vi "menuSelection.vi"(8 "error in (no error)":errorcluster, 9 "MenuRef":refnum<k9>, 10 "itemPath":string, 11 "ImageStreamViewer in":refnum<class "ImageStreamViewer.lvclass">) -> (0 "error out":errorcluster, 2 "close":bool, 3 "ImageStreamViewer out":refnum<class "ImageStreamViewer.lvclass">)   [LabVIEW 2011, in "Views.lvlib" / "Camera.lvlib" / "ImageStreamViewer.lvclass"]
uses:
  ImageStreamViewer.lvclass
  Tools/ImageProcessor/ImageAnalyser/AbsorptionAnalyser/AbsorptionAnalyser.lvclass
  Tools/ImageProcessor/ImageAnalyser/AbsorptionDS/AbsorptionDS.lvclass
  Tools/ImageProcessor/ImageAnalyser/FluorescenceAnalyser/FluorescenceAnalyser.lvclass
  Tools/ImageProcessor/ImageAnalyser/FluorescenceLiveAnalyser/FluorescenceLiveAnalyser.lvclass
  Tools/ImageProcessor/ImageAnalyser/TemperatureAnalyser/TemperatureAnalyser.lvclass
  Tools/ImageProcessor/ImageAnalyser/FringeTesting/FringeTesting.lvclass
  Tools/ImageProcessor/ImageAnalyser/Absorption2/Absorption2.lvclass
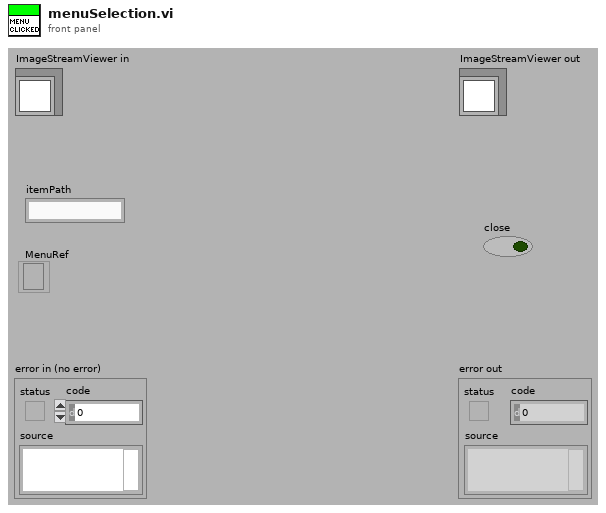
[diagram p1: front panel]
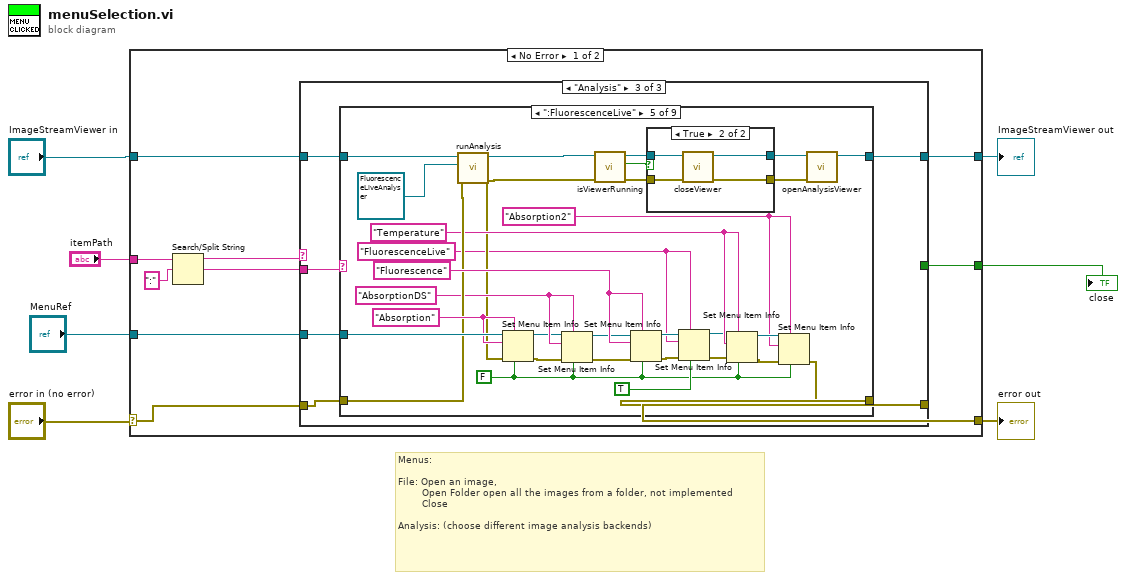
[diagram p0: block diagram]
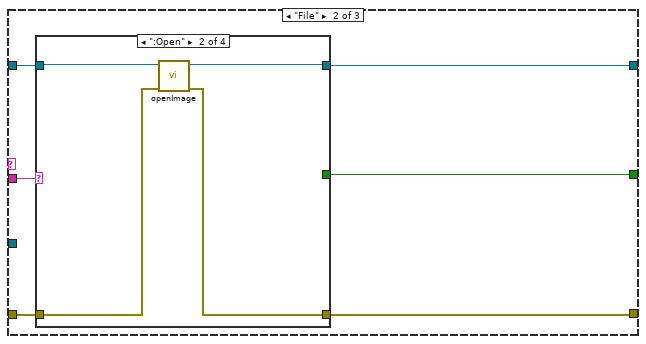
[diagram p3: hidden frame]
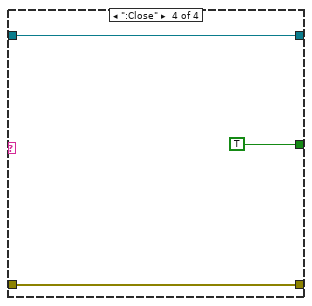
[diagram p6: hidden frame]
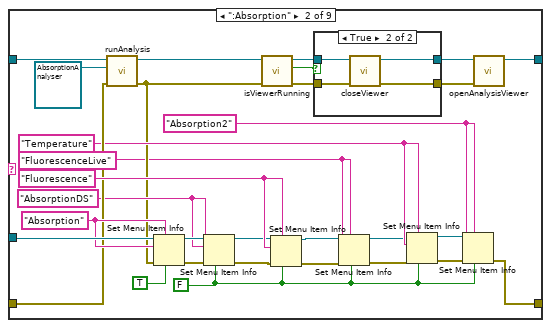
[diagram p8: hidden frame]
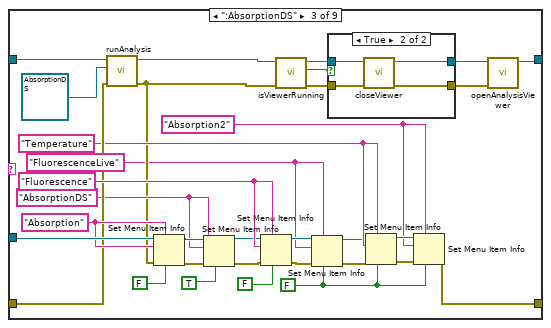
[diagram p10: hidden frame]
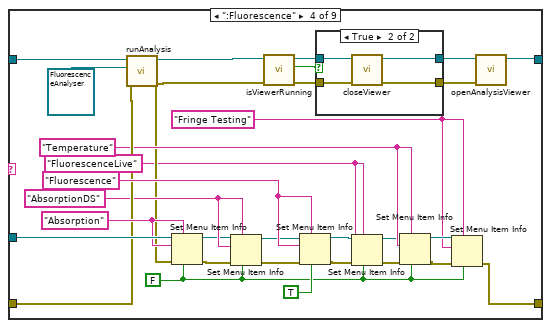
[diagram p12: hidden frame]
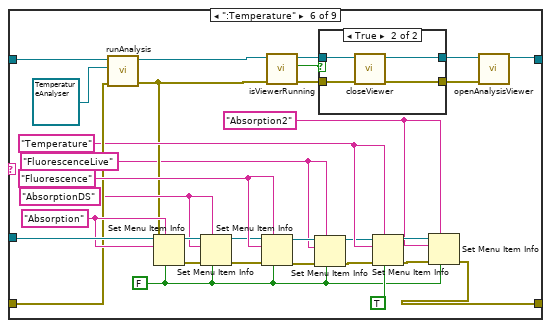
[diagram p15: hidden frame]
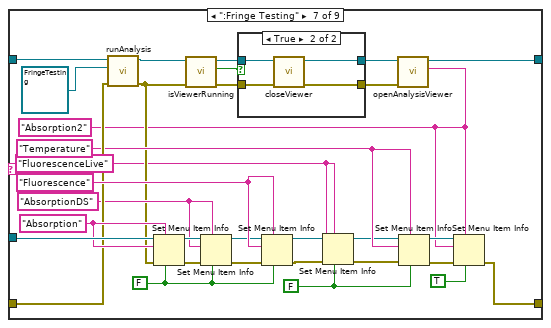
[diagram p17: hidden frame]
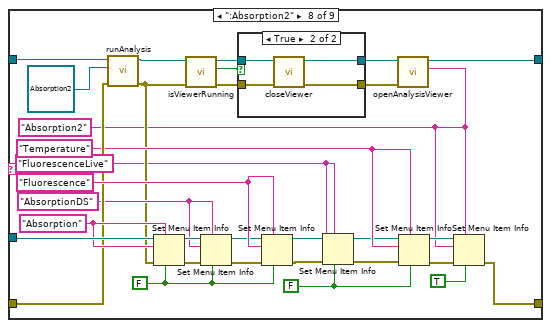
[diagram p19: hidden frame]
diagram:
  # "Menus: \n\nFile: Open an image, \n        Open Folder open all the images from a folder, not implemented\n        Close\n\nAnalysis: (choose different image analysis backends)"
  n1 = case shown="No Error" "error in (no error)" {
    selector: "error in (no error)" -> [w16 w313]
    tunnel: [w15 w313] -> w1
    tunnel: [w12 w312] -> w5
    tunnel: "ImageStreamViewer in" -> [w11 w312]
    tunnel: [w10 _] -> w6
    tunnel: "itemPath" -> [w9 _]
    tunnel: "MenuRef" -> [w8 _]
    frame No Error {
      n2 = Search/Split String(string=w9, search string/char (-)=":") -> (substring before match=w14:string, match + rest of string=w13:string)  [unwired: 1 in, 1 out]
      n3 = case shown="\"Analysis\"" w14 {
        tunnel: w16 -> [w18 w25 w39]
        tunnel: [w18 w24 w38] -> w15
        tunnel: w13 -> [_ w21 w40]
        tunnel: w11 -> [w19 w23 w42]
        tunnel: [w19 w22 w41] -> w12
        tunnel: [_ w20 _] -> w10
        tunnel: w8 -> [_ _ w37]
        frame Default {
        }
        frame "File" {
          n4 = case shown="\":Open\"" w21 {
            tunnel: w25 -> [w26 w29 w32 w35]
            tunnel: [w26 w28 w32 w35] -> w24
            tunnel: w23 -> [w27 w31 w33 w36]
            tunnel: [w27 w30 w33 w36] -> w22
            tunnel: [_ _ _ TRUE] -> w20
            frame Default {
            }
            frame ":Open" {
              n5 = call "openImage.vi"("error in (no error)"=w29, "ImageStreamViewer in"=w31) -> ("error out"=w28:errorcluster, "ImageStreamViewer out"=w30:refnum<class "ImageStreamViewer.lvclass">)  [unwired: 8 in]
            }
            frame ":Open Folder" {
            }
            frame ":Close" {
            }
          }
        }
        frame "Analysis" {
          n6 = case shown="\":FluorescenceLive\"" w40 {
            tunnel: w42 -> [w44 w71 w109 w148 w185 w222 w260 w298 w311]
            tunnel: [w44 w51 w88 w127 w166 w201 w239 w278 w310] -> w41
            tunnel: w39 -> [w43 w70 w108 w147 w184 w221 w259 w297 w309]
            tunnel: [w43 w59 w97 w136 w175 w210 w248 w286 w308] -> w38
            tunnel: w37 -> [_ w75 w114 w151 w188 w225 w263 w301 _]
            frame Default {
            }
            frame ":Absorption" {
              w46 = "FluorescenceLive"
              w60 = "Absorption2"
              w63 = "AbsorptionDS"
              w68 = "Temperature"
              w73 = "Absorption"
              w72 = "Fluorescence"
              w45 = FALSE
              n7 = call "runAnalysis.vi"("error in (no error)"=w70, "ImageAnalyser"=refnum<class "AbsorptionAnalyser.lvclass"> refnum ("Tools.lvlib:Imaging.lvlib:AbsorptionAnalyser.lvclass"), "ImageStreamViewer in"=w71) -> ("error out"=w52:errorcluster, "ImageStreamViewer out"=w53:refnum<class "ImageStreamViewer.lvclass">)  [unwired: 7 in]
              n8 = Set Menu Item Info(6:TRUE, 7:w73, 8:w52, 10:w73, 11:w75) -> (0:w65:errorcluster, 3:w67:refnum<k9>)  [unwired: 2 in]
              n9 = Set Menu Item Info(6:w45, 7:w63, 8:w65, 10:w63, 11:w67) -> (0:w64:errorcluster, 3:w66:refnum<k9>)  [unwired: 2 in]
              n10 = call "isViewerRunning.vi"("error in (no error)"=w52, "ImageStreamViewer in"=w53) -> ("error out"=w57:errorcluster, "running?"=w56:bool, "ImageStreamViewer out"=w58:refnum<class "ImageStreamViewer.lvclass">)  [unwired: 7 in]
              n11 = Set Menu Item Info(6:w45, 7:w72, 8:w64, 10:w72, 11:w66) -> (0:w48:errorcluster, 3:w50:refnum<k9>)  [unwired: 2 in]
              n12 = case shown="True" w56 {
                tunnel: w58 -> [w77 w81]
                tunnel: w57 -> [w76 w80]
                tunnel: [w77 w79] -> w55
                tunnel: [w76 w78] -> w54
                frame False {
                }
                frame True {
                  n13 = call "closeViewer.vi"("error in (no error)"=w80, "ImageStreamViewer in"=w81) -> ("error out"=w78:errorcluster, "ImageStreamViewer out"=w79:refnum<class "ImageStreamViewer.lvclass">)  [unwired: 8 in]
                }
              }
              n14 = Set Menu Item Info(6:w45, 7:w46, 8:w48, 10:w46, 11:w50) -> (0:w47:errorcluster, 3:w49:refnum<k9>)  [unwired: 2 in]
              n15 = Set Menu Item Info(6:w45, 7:w68, 8:w47, 10:w68, 11:w49) -> (0:w61:errorcluster, 3:w62:refnum<k9>)  [unwired: 2 in]
              n16 = Set Menu Item Info(6:w45, 7:w60, 8:w61, 10:w60, 11:w62) -> (0:w59:errorcluster)  [unwired: 2 in, 1 out]
              n17 = call "openAnalysisViewer.vi"("error in (no error)"=w54, "ImageStreamViewer in"=w55) -> ("ImageStreamViewer out"=w51:refnum<class "ImageStreamViewer.lvclass">)  [unwired: 8 in, 1 out]
            }
            frame ":AbsorptionDS" {
              w83 = "FluorescenceLive"
              w96 = "Absorption2"
              w100 = "AbsorptionDS"
              w107 = "Temperature"
              w82 = FALSE
              w111 = "Absorption"
              w110 = "Fluorescence"
              n18 = call "runAnalysis.vi"("error in (no error)"=w108, "ImageAnalyser"=refnum<class "AbsorptionDS.lvclass"> refnum ("Tools.lvlib:Imaging.lvlib:AbsorptionDS.lvclass"), "ImageStreamViewer in"=w109) -> ("error out"=w89:errorcluster, "ImageStreamViewer out"=w90:refnum<class "ImageStreamViewer.lvclass">)  [unwired: 7 in]
              n19 = Set Menu Item Info(6:FALSE, 7:w111, 8:w89, 10:w111, 11:w114) -> (0:w103:errorcluster, 3:w104:refnum<k9>)  [unwired: 2 in]
              n20 = Set Menu Item Info(6:TRUE, 7:w100, 8:w103, 10:w100, 11:w104) -> (0:w102:errorcluster, 3:w105:refnum<k9>)  [unwired: 2 in]
              n21 = Set Menu Item Info(6:FALSE, 7:w110, 8:w102, 10:w110, 11:w105) -> (0:w86:errorcluster, 3:w87:refnum<k9>)  [unwired: 2 in]
              n22 = call "isViewerRunning.vi"("error in (no error)"=w89, "ImageStreamViewer in"=w90) -> ("error out"=w94:errorcluster, "running?"=w93:bool, "ImageStreamViewer out"=w95:refnum<class "ImageStreamViewer.lvclass">)  [unwired: 7 in]
              n23 = Set Menu Item Info(6:w82, 7:w83, 8:w86, 10:w83, 11:w87) -> (0:w85:errorcluster, 3:w84:refnum<k9>)  [unwired: 2 in]
              n24 = case shown="True" w93 {
                tunnel: w95 -> [w116 w120]
                tunnel: w94 -> [w115 w119]
                tunnel: [w116 w118] -> w92
                tunnel: [w115 w117] -> w91
                frame False {
                }
                frame True {
                  n25 = call "closeViewer.vi"("error in (no error)"=w119, "ImageStreamViewer in"=w120) -> ("error out"=w117:errorcluster, "ImageStreamViewer out"=w118:refnum<class "ImageStreamViewer.lvclass">)  [unwired: 8 in]
                }
              }
              n26 = Set Menu Item Info(6:w82, 7:w107, 8:w85, 10:w107, 11:w84) -> (0:w98:errorcluster, 3:w99:refnum<k9>)  [unwired: 2 in]
              n27 = Set Menu Item Info(6:w82, 7:w96, 8:w98, 10:w96, 11:w99) -> (0:w97:errorcluster)  [unwired: 2 in, 1 out]
              n28 = call "openAnalysisViewer.vi"("error in (no error)"=w91, "ImageStreamViewer in"=w92) -> ("ImageStreamViewer out"=w88:refnum<class "ImageStreamViewer.lvclass">)  [unwired: 8 in, 1 out]
            }
            frame ":Fluorescence" {
              w121 = "FluorescenceLive"
              w135 = "Fringe Testing"
              w144 = "AbsorptionDS"
              w145 = "Temperature"
              w150 = "Absorption"
              w149 = "Fluorescence"
              w122 = FALSE
              n29 = call "runAnalysis.vi"("error in (no error)"=w147, "ImageAnalyser"=refnum<class "FluorescenceAnalyser.lvclass"> refnum ("Tools.lvlib:Imaging.lvlib:FluorescenceAnalyser.lvclass"), "ImageStreamViewer in"=w148) -> ("error out"=w128:errorcluster, "ImageStreamViewer out"=w129:refnum<class "ImageStreamViewer.lvclass">)  [unwired: 7 in]
              n30 = Set Menu Item Info(6:w122, 7:w150, 8:w128, 10:w150, 11:w151) -> (0:w141:errorcluster, 3:w143:refnum<k9>)  [unwired: 2 in]
              n31 = Set Menu Item Info(6:w122, 7:w144, 8:w141, 10:w144, 11:w143) -> (0:w140:errorcluster, 3:w142:refnum<k9>)  [unwired: 2 in]
              n32 = call "isViewerRunning.vi"("error in (no error)"=w128, "ImageStreamViewer in"=w129) -> ("error out"=w133:errorcluster, "running?"=w132:bool, "ImageStreamViewer out"=w134:refnum<class "ImageStreamViewer.lvclass">)  [unwired: 7 in]
              n33 = Set Menu Item Info(6:TRUE, 7:w149, 8:w140, 10:w149, 11:w142) -> (0:w123:errorcluster, 3:w126:refnum<k9>)  [unwired: 2 in]
              n34 = case shown="True" w132 {
                tunnel: w134 -> [w153 w157]
                tunnel: w133 -> [w152 w156]
                tunnel: [w153 w155] -> w131
                tunnel: [w152 w154] -> w130
                frame False {
                }
                frame True {
                  n35 = call "closeViewer.vi"("error in (no error)"=w156, "ImageStreamViewer in"=w157) -> ("error out"=w154:errorcluster, "ImageStreamViewer out"=w155:refnum<class "ImageStreamViewer.lvclass">)  [unwired: 8 in]
                }
              }
              n36 = Set Menu Item Info(6:w122, 7:w121, 8:w123, 10:w121, 11:w126) -> (0:w124:errorcluster, 3:w125:refnum<k9>)  [unwired: 2 in]
              n37 = Set Menu Item Info(6:w122, 7:w145, 8:w124, 10:w145, 11:w125) -> (0:w137:errorcluster, 3:w138:refnum<k9>)  [unwired: 2 in]
              n38 = Set Menu Item Info(6:w122, 7:w135, 8:w137, 10:w135, 11:w138) -> (0:w136:errorcluster)  [unwired: 2 in, 1 out]
              n39 = call "openAnalysisViewer.vi"("error in (no error)"=w130, "ImageStreamViewer in"=w131) -> ("ImageStreamViewer out"=w127:refnum<class "ImageStreamViewer.lvclass">)  [unwired: 8 in, 1 out]
            }
            frame ":FluorescenceLive" {
              w160 = "FluorescenceLive"
              w174 = "Absorption2"
              w182 = "AbsorptionDS"
              w183 = "Temperature"
              w187 = "Absorption"
              w186 = "Fluorescence"
              w158 = FALSE
              n40 = call "runAnalysis.vi"("error in (no error)"=w184, "ImageAnalyser"=refnum<class "FluorescenceLiveAnalyser.lvclass"> refnum ("Tools.lvlib:Imaging.lvlib:FluorescenceLiveAnalyser.lvclass"), "ImageStreamViewer in"=w185) -> ("error out"=w167:errorcluster, "ImageStreamViewer out"=w168:refnum<class "ImageStreamViewer.lvclass">)  [unwired: 7 in]
              n41 = Set Menu Item Info(6:w158, 7:w187, 8:w167, 10:w187, 11:w188) -> (0:w179:errorcluster, 3:w181:refnum<k9>)  [unwired: 2 in]
              n42 = Set Menu Item Info(6:w158, 7:w182, 8:w179, 10:w182, 11:w181) -> (0:w178:errorcluster, 3:w180:refnum<k9>)  [unwired: 2 in]
              n43 = call "isViewerRunning.vi"("error in (no error)"=w167, "ImageStreamViewer in"=w168) -> ("error out"=w172:errorcluster, "running?"=w171:bool, "ImageStreamViewer out"=w173:refnum<class "ImageStreamViewer.lvclass">)  [unwired: 7 in]
              n44 = Set Menu Item Info(6:w158, 7:w186, 8:w178, 10:w186, 11:w180) -> (0:w163:errorcluster, 3:w164:refnum<k9>)  [unwired: 2 in]
              n45 = case shown="True" w171 {
                tunnel: w173 -> [w190 w194]
                tunnel: w172 -> [w189 w193]
                tunnel: [w190 w192] -> w170
                tunnel: [w189 w191] -> w169
                frame False {
                }
                frame True {
                  n46 = call "closeViewer.vi"("error in (no error)"=w193, "ImageStreamViewer in"=w194) -> ("error out"=w191:errorcluster, "ImageStreamViewer out"=w192:refnum<class "ImageStreamViewer.lvclass">)  [unwired: 8 in]
                }
              }
              n47 = Set Menu Item Info(6:TRUE, 7:w160, 8:w163, 10:w160, 11:w164) -> (0:w162:errorcluster, 3:w161:refnum<k9>)  [unwired: 2 in]
              n48 = Set Menu Item Info(6:w158, 7:w183, 8:w162, 10:w183, 11:w161) -> (0:w176:errorcluster, 3:w177:refnum<k9>)  [unwired: 2 in]
              n49 = Set Menu Item Info(6:w158, 7:w174, 8:w176, 10:w174, 11:w177) -> (0:w175:errorcluster)  [unwired: 2 in, 1 out]
              n50 = call "openAnalysisViewer.vi"("error in (no error)"=w169, "ImageStreamViewer in"=w170) -> ("ImageStreamViewer out"=w166:refnum<class "ImageStreamViewer.lvclass">)  [unwired: 8 in, 1 out]
            }
            frame ":Temperature" {
              w196 = "FluorescenceLive"
              w209 = "Absorption2"
              w213 = "AbsorptionDS"
              w219 = "Temperature"
              w224 = "Absorption"
              w223 = "Fluorescence"
              w195 = FALSE
              n51 = call "runAnalysis.vi"("error in (no error)"=w221, "ImageAnalyser"=refnum<class "TemperatureAnalyser.lvclass"> refnum ("Tools.lvlib:Imaging.lvlib:TemperatureAnalyser.lvclass"), "ImageStreamViewer in"=w222) -> ("error out"=w202:errorcluster, "ImageStreamViewer out"=w203:refnum<class "ImageStreamViewer.lvclass">)  [unwired: 7 in]
              n52 = Set Menu Item Info(6:w195, 7:w224, 8:w202, 10:w224, 11:w225) -> (0:w215:errorcluster, 3:w217:refnum<k9>)  [unwired: 2 in]
              n53 = Set Menu Item Info(6:w195, 7:w213, 8:w215, 10:w213, 11:w217) -> (0:w214:errorcluster, 3:w216:refnum<k9>)  [unwired: 2 in]
              n54 = Set Menu Item Info(6:w195, 7:w223, 8:w214, 10:w223, 11:w216) -> (0:w197:errorcluster, 3:w200:refnum<k9>)  [unwired: 2 in]
              n55 = call "isViewerRunning.vi"("error in (no error)"=w202, "ImageStreamViewer in"=w203) -> ("error out"=w207:errorcluster, "running?"=w206:bool, "ImageStreamViewer out"=w208:refnum<class "ImageStreamViewer.lvclass">)  [unwired: 7 in]
              n56 = Set Menu Item Info(6:w195, 7:w196, 8:w197, 10:w196, 11:w200) -> (0:w198:errorcluster, 3:w199:refnum<k9>)  [unwired: 2 in]
              n57 = case shown="True" w206 {
                tunnel: w208 -> [w227 w231]
                tunnel: w207 -> [w226 w230]
                tunnel: [w227 w229] -> w205
                tunnel: [w226 w228] -> w204
                frame False {
                }
                frame True {
                  n58 = call "closeViewer.vi"("error in (no error)"=w230, "ImageStreamViewer in"=w231) -> ("error out"=w228:errorcluster, "ImageStreamViewer out"=w229:refnum<class "ImageStreamViewer.lvclass">)  [unwired: 8 in]
                }
              }
              n59 = Set Menu Item Info(6:TRUE, 7:w219, 8:w198, 10:w219, 11:w199) -> (0:w211:errorcluster, 3:w212:refnum<k9>)  [unwired: 2 in]
              n60 = Set Menu Item Info(6:w195, 7:w209, 8:w211, 10:w209, 11:w212) -> (0:w210:errorcluster)  [unwired: 2 in, 1 out]
              n61 = call "openAnalysisViewer.vi"("error in (no error)"=w204, "ImageStreamViewer in"=w205) -> ("ImageStreamViewer out"=w201:refnum<class "ImageStreamViewer.lvclass">)  [unwired: 8 in, 1 out]
            }
            frame ":Fringe Testing" {
              w233 = "FluorescenceLive"
              w238 = "Absorption2"
              w252 = "AbsorptionDS"
              w232 = FALSE
              w258 = "Temperature"
              w262 = "Absorption"
              w261 = "Fluorescence"
              w253 = FALSE
              n62 = call "runAnalysis.vi"("error in (no error)"=w259, "ImageAnalyser"=refnum<class "FringeTesting.lvclass"> refnum ("Tools.lvlib:Imaging.lvlib:FringeTesting.lvclass"), "ImageStreamViewer in"=w260) -> ("error out"=w245:errorcluster, "ImageStreamViewer out"=w246:refnum<class "ImageStreamViewer.lvclass">)  [unwired: 7 in]
              n63 = Set Menu Item Info(6:w253, 7:w262, 8:w245, 10:w262, 11:w263) -> (0:w255:errorcluster, 3:w257:refnum<k9>)  [unwired: 2 in]
              n64 = call "isViewerRunning.vi"("error in (no error)"=w245, "ImageStreamViewer in"=w246) -> ("error out"=w243:errorcluster, "running?"=w242:bool, "ImageStreamViewer out"=w244:refnum<class "ImageStreamViewer.lvclass">)  [unwired: 7 in]
              n65 = Set Menu Item Info(6:w253, 7:w252, 8:w255, 10:w252, 11:w257) -> (0:w254:errorcluster, 3:w256:refnum<k9>)  [unwired: 2 in]
              n66 = case shown="True" w242 {
                tunnel: w244 -> [w265 w269]
                tunnel: w243 -> [w264 w268]
                tunnel: [w265 w267] -> w241
                tunnel: [w264 w266] -> w240
                frame False {
                }
                frame True {
                  n67 = call "closeViewer.vi"("error in (no error)"=w268, "ImageStreamViewer in"=w269) -> ("error out"=w266:errorcluster, "ImageStreamViewer out"=w267:refnum<class "ImageStreamViewer.lvclass">)  [unwired: 8 in]
                }
              }
              n68 = Set Menu Item Info(6:w253, 7:w261, 8:w254, 10:w261, 11:w256) -> (0:w236:errorcluster, 3:w237:refnum<k9>)  [unwired: 2 in]
              n69 = Set Menu Item Info(6:w232, 7:w233, 8:w236, 10:w233, 11:w237) -> (0:w235:errorcluster, 3:w234:refnum<k9>)  [unwired: 2 in]
              n70 = call "openAnalysisViewer.vi"("error in (no error)"=w240, "whichViewer"=w238, "ImageStreamViewer in"=w241) -> ("ImageStreamViewer out"=w239:refnum<class "ImageStreamViewer.lvclass">)  [unwired: 7 in, 1 out]
              n71 = Set Menu Item Info(6:w232, 7:w258, 8:w235, 10:w258, 11:w234) -> (0:w250:errorcluster, 3:w251:refnum<k9>)  [unwired: 2 in]
              n72 = Set Menu Item Info(6:TRUE, 7:w238, 8:w250, 10:w238, 11:w251) -> (0:w248:errorcluster)  [unwired: 2 in, 1 out]
            }
            frame ":Absorption2" {
              w272 = "FluorescenceLive"
              w277 = "Absorption2"
              w290 = "AbsorptionDS"
              w271 = FALSE
              w296 = "Temperature"
              w300 = "Absorption"
              w299 = "Fluorescence"
              w291 = FALSE
              n73 = call "runAnalysis.vi"("error in (no error)"=w297, "ImageAnalyser"=refnum<class "Absorption2.lvclass"> refnum ("Tools.lvlib:Imaging.lvlib:Absorption2.lvclass"), "ImageStreamViewer in"=w298) -> ("error out"=w284:errorcluster, "ImageStreamViewer out"=w285:refnum<class "ImageStreamViewer.lvclass">)  [unwired: 7 in]
              n74 = Set Menu Item Info(6:w291, 7:w300, 8:w284, 10:w300, 11:w301) -> (0:w293:errorcluster, 3:w295:refnum<k9>)  [unwired: 2 in]
              n75 = call "isViewerRunning.vi"("error in (no error)"=w284, "ImageStreamViewer in"=w285) -> ("error out"=w282:errorcluster, "running?"=w281:bool, "ImageStreamViewer out"=w283:refnum<class "ImageStreamViewer.lvclass">)  [unwired: 7 in]
              n76 = Set Menu Item Info(6:w291, 7:w290, 8:w293, 10:w290, 11:w295) -> (0:w292:errorcluster, 3:w294:refnum<k9>)  [unwired: 2 in]
              n77 = case shown="True" w281 {
                tunnel: w283 -> [w303 w307]
                tunnel: w282 -> [w302 w306]
                tunnel: [w303 w305] -> w280
                tunnel: [w302 w304] -> w279
                frame False {
                }
                frame True {
                  n78 = call "closeViewer.vi"("error in (no error)"=w306, "ImageStreamViewer in"=w307) -> ("error out"=w304:errorcluster, "ImageStreamViewer out"=w305:refnum<class "ImageStreamViewer.lvclass">)  [unwired: 8 in]
                }
              }
              n79 = Set Menu Item Info(6:w291, 7:w299, 8:w292, 10:w299, 11:w294) -> (0:w275:errorcluster, 3:w276:refnum<k9>)  [unwired: 2 in]
              n80 = Set Menu Item Info(6:w271, 7:w272, 8:w275, 10:w272, 11:w276) -> (0:w274:errorcluster, 3:w273:refnum<k9>)  [unwired: 2 in]
              n81 = call "openAnalysisViewer.vi"("error in (no error)"=w279, "whichViewer"=w277, "ImageStreamViewer in"=w280) -> ("ImageStreamViewer out"=w278:refnum<class "ImageStreamViewer.lvclass">)  [unwired: 7 in, 1 out]
              n82 = Set Menu Item Info(6:w271, 7:w296, 8:w274, 10:w296, 11:w273) -> (0:w288:errorcluster, 3:w289:refnum<k9>)  [unwired: 2 in]
              n83 = Set Menu Item Info(6:TRUE, 7:w277, 8:w288, 10:w277, 11:w289) -> (0:w286:errorcluster)  [unwired: 2 in, 1 out]
            }
            frame ":Show Analysis Viewer" {
              n84 = call "showAnalysisViewer.vi"("error in (no error)"=w309, "ImageStreamViewer in"=w311) -> ("error out"=w308:errorcluster, "ImageStreamViewer out"=w310:refnum<class "ImageStreamViewer.lvclass">)  [unwired: 8 in]
            }
          }
        }
      }
    }
    frame Error {
    }
  }
  "error out" <- w1
  "ImageStreamViewer out" <- w5
  "close" <- w6
